vi "Set Speed or Torque.vi"(6 "Control Mode":u8(ring)=2 items=["Velocity"=2, "Torque"=1], 7 "timeout (1s)":dbl=1.0 min=0.0, 8 "error in (no error)":errorcluster, 9 "Speed":i32(knob) scale=0.0..4000.0, 10 "Torque":i16(knob) scale=-200.0..200.0, 11 "SDO object in":refnum<k20>) -> (0 "error out":errorcluster, 1 "completion code":u32, 3 "SDO object out":refnum<k20>)   [LabVIEW 2016]
uses:
  Set target torque.vi
  Set target speed.vi
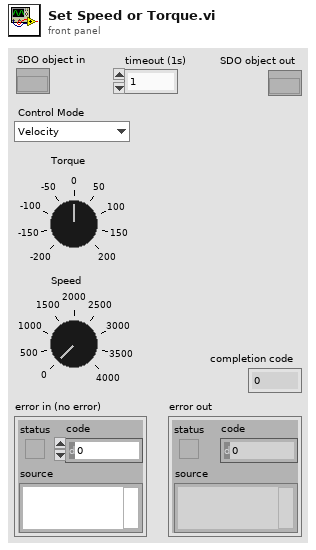
[diagram p1: front panel]
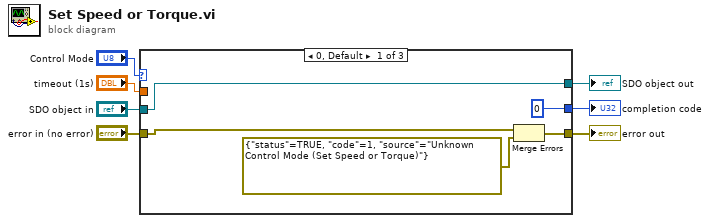
[diagram p0: block diagram]
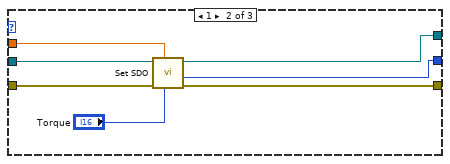
[diagram p2: hidden frame]
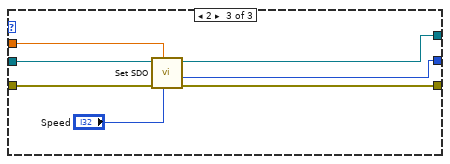
[diagram p3: hidden frame]
diagram:
  n1 = case shown="0, Default" "Control Mode" {
    tunnel: "error in (no error)" -> [w10 w19 w26]
    tunnel: "SDO object in" -> [w8 w18 w25]
    tunnel: [w8 w16 w24] -> w4
    tunnel: [w12 w15 w23] -> w3
    tunnel: "timeout (1s)" -> [_ w17 w22]
    tunnel: [u32 0 ("completion code") w14 w21] -> w1
    frame 0, Default {
      n2 = Merge Errors(w10, errorcluster {"status"=TRUE, "code"=1, "source"="Unknown Control Mode (Set Speed or Torque)"} ("error constant")) -> (w12:errorcluster)
    }
    frame 1 {
      n3 = call-poly "Set SDO.vi"("Torque"="Torque", "timeout (1s)"=w17, "error in (no error)"=w19, "SDO object in"=w18) -> ("error out"=w15:errorcluster, "completion code"=w14:u32, "SDO object out"=w16:refnum<k20>)  [unwired: 5 in]
    }
    frame 2 {
      n4 = call-poly "Set SDO.vi"("Speed"="Speed", "timeout (1s)"=w22, "error in (no error)"=w26, "SDO object in"=w25) -> ("error out"=w23:errorcluster, "completion code"=w21:u32, "SDO object out"=w24:refnum<k20>)  [unwired: 5 in]
    }
  }
  "SDO object out" <- w4
  "completion code" <- w1
  "error out" <- w3
